vi "Handle Camera Configuration.vi"(9 "CameraNameRef":refnum<vi>, 10 "Display Name":string="Camera", 11 "ClusterRef":refnum<vi>) -> ()   [LabVIEW 2017]
uses:
  <vilib>/Rock Robotics/Network Tables/Make Table Operation.ctl
  <vilib>/Utility/config.llb/Read Key (String).vi
  <vilib>/Utility/config.llb/Read Key (I32).vi
  <vilib>/Utility/config.llb/Write Key (String).vi
  <vilib>/Utility/config.llb/Write Key (I32).vi
  <vilib>/Utility/config.llb/NI_LVConfig.lvlib
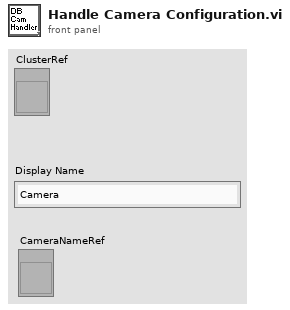
[diagram p1: front panel]
types:
  T1 = typedef "NI_LVConfig.lvlib/Config Data RefNum.ctl" = refnum<k1>
  T2 = cluster{"value":i32, "value":i32, "index":i32, bool}
  T3 = typedef "Make Table Operation.ctl" = enum16{"Get or Add Field", "Get Field or Add Temp", "Replace Temp ID", "Get Field ID - No Add", "Get Table Field IDs", "Get Field ID Info", "Move Field to Temp", "Validate", "Remove Field", "Remove All"}
  T4 = cluster{"Frame Rate":i32, "Compression":i32, "Size":u16, "DB Camera Config":bool}
  T5 = typedef "Field ID.ctl" = i32
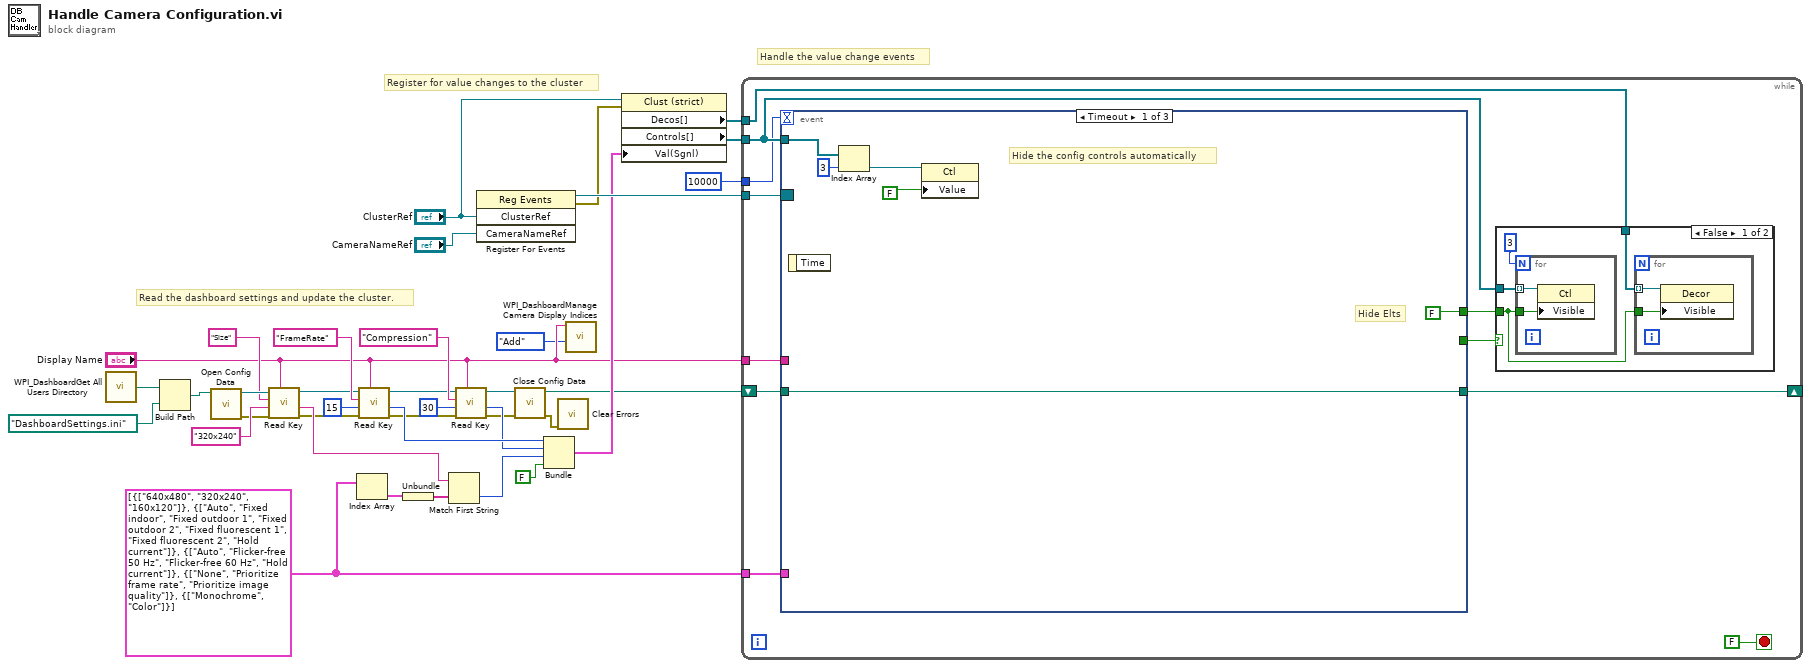
[diagram p0: block diagram]
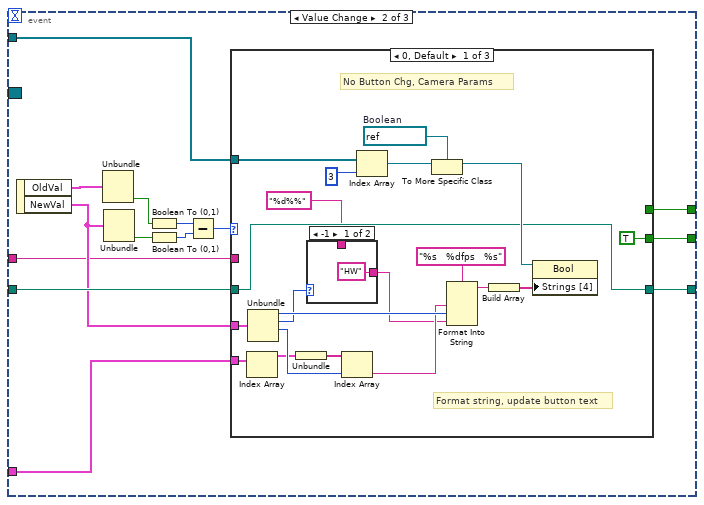
[diagram p3: hidden frame]
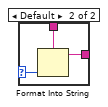
[diagram p4: hidden frame]
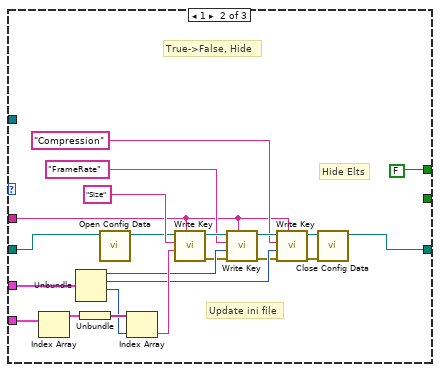
[diagram p5: hidden frame]
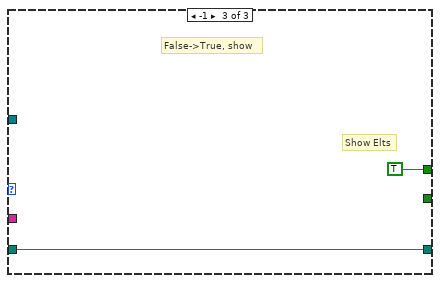
[diagram p6: hidden frame]
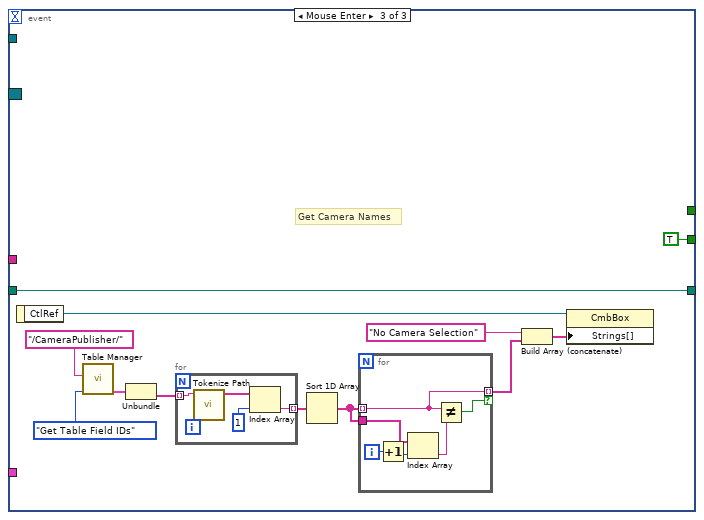
[diagram p7: hidden frame]
diagram:
  w16 = cluster{string[]}[] [{["640x480", "320x240", "160x120"]}, {["Auto", "Fixed indoor", "Fixed outdoor 1", "Fixed outdoor 2", "Fixed fluorescent 1", "Fixed fluorescent 2", "Hold current"]}, {["Auto", "Flicker-free 50 Hz", "Flicker-free 60 Hz", "Hold current"]}, {["None", "Prioritize frame rate", "Prioritize image quality"]}, {["Monochrome", "Color"]}]
  # "Handle the value change events"
  # "Register for value changes to the cluster"
  # "Read the dashboard settings and update the cluster."
  n1 = call <vilib>:"WPI_DashboardGet All Users Directory.vi"() -> ("All User Path"=w34:path)
  n2 = Build Path(base path=w34, name or relative path=path "DashboardSettings.ini") -> (appended path=w33:path)
  n3 = call <vilib>:"Open Config Data.vi"("configuration file path"=w33) -> ("error out"=w10:errorcluster, "refnum"=w32:T1)  [unwired: 8 in, 1 out]
  n4 = call-poly <vilib>:"Read Key.vi"("section"="Display Name", "error in (no error)"=w10, "default value"="320x240", "key"="Size", "refnum"=w32) -> ("error out"=w9:errorcluster, "value"=w20:string, "refnum out"=w24:T1)  [unwired: 1 in, 3 out]
  n5 = Index Array(array=w16) -> (element=w22:cluster{string[]})  [unwired: 1 in]
  n6 = call-poly <vilib>:"Read Key.vi"("section"="Display Name", "error in (no error)"=w9, "default value"=15, "key"="FrameRate", "refnum"=w24) -> ("error out"=w8:errorcluster, "value"=w18:i32, "refnum out"=w23:T1)  [unwired: 4 out]
  n7 = Unbundle(w22) -> (w21:string[])
  n8 = Match First String(2:w21, 3:w20) -> (0:w19:i32)  [unwired: 1 out]
  n9 = call-poly <vilib>:"Read Key.vi"("section"="Display Name", "error in (no error)"=w8, "default value"=30, "key"="Compression", "refnum"=w23) -> ("error out"=w5:errorcluster, "value"=w17:i32, "refnum out"=w7:T1)  [unwired: 4 out]
  n10 = register-events("ClusterRef", "CameraNameRef") -> (reference out=w37:refnum<event-registration>, error out=w14:errorcluster)  [unwired: 2 in]
  n11 = call <vilib>:"Close Config Data.vi"("error in (no error)"=w5, "refnum"=w7) -> ("error out"=w4:errorcluster, "file path"=w6:path)  [unwired: 1 in, 7 out]
  n12 = Bundle("value"=w18, "value"=w17, "index"=w19, FALSE) -> (w13:T2)  [unwired: 1 out]
  n13 = call <vilib>:"Clear Errors.vi"("error in (no error)"=w4) -> ()  [unwired: 5 in, 2 out]
  n14 = call <vilib>:"WPI_DashboardManage Camera Display Indices.vi"("Operation"=enum16{"Add", "Retrieve"}."Add", "Display Name"="Display Name") -> ()  [unwired: 9 in, 1 out]
  n15 = property class="Clust (strict)"(reference="ClusterRef", error in=w14, "Val(Sgnl)"=w13) -> ("Decos[]"=w12:refnum<vi>[], "Controls[]"=w35:refnum<vi>[])  [unwired: 2 out]
  n16 = while {
    tunnel: w37 -> [w48]
    tunnel: w35 -> [w40]
    shift-right: [w46] -> _
    shift-left: w6 -> [w47]
    tunnel: w16 -> [w45]
    tunnel: "Display Name" -> [w43]
    tunnel: w12 -> [w39]
    tunnel: 10000 -> [w38]
    stop <- FALSE stop-if-true
    n17 = event shown="[0] Timeout" {
      selector: w48 -> [_ _ _]
      dyn-events: _ -> [_ _ _]
      timeout: w38 -> [_ _ _]
      tunnel: w47 -> [w61 w70 w134]
      tunnel: [w61 w66 w134] -> w46
      tunnel: w45 -> [_ w68 _]
      tunnel: w40 -> [w60 w67 _]
      tunnel: w43 -> [_ w65 _]
      tunnel: [FALSE w64 _] -> w41
      tunnel: [_ w63 TRUE] -> w42
      event Timeout {
        # "Hide Elts"
        # "Hide the config controls automatically"
        n18 = event-data() -> ()  [unwired: 1 in, 1 out]
        n19 = Index Array(array=w60, index=3) -> (element=w58:refnum<vi>)
        n20 = property class="Ctl"(reference=w58, "Value"=FALSE) -> ()  [unwired: 1 in, 2 out]
      }
      event Value Change {
        n21 = event-data() -> ("OldVal"=w72:T4, "NewVal"=w69:T4)  [unwired: 1 in]
        n22 = Unbundle(w72) -> ("DB Camera Config"=w76:bool)  [unwired: 3 out]
        n23 = Unbundle(w69) -> ("DB Camera Config"=w75:bool)  [unwired: 3 out]
        n24 = Boolean To (0,1)(Boolean=w76) -> (0, 1=w73:i16)
        n25 = Boolean To (0,1)(Boolean=w75) -> (0, 1=w74:i16)
        n26 = Subtract(x=w73, y=w74) -> (x-y=w71:i16)
        n27 = case shown="0, Default" w71 {
          tunnel: [_ FALSE TRUE] -> w64
          tunnel: [TRUE _ _] -> w63
          tunnel: w70 -> [w80 w103 w123]
          tunnel: w69 -> [w88 w112 _]
          tunnel: w68 -> [w87 w108 _]
          tunnel: w67 -> [w86 _ _]
          tunnel: [w80 w101 w123] -> w66
          tunnel: w65 -> [_ w107 _]
          frame 0, Default {
            w83 = refnum<vi> refnum  # Boolean
            # "Format string, update button text"
            # "No Button Chg, Camera Params"
            n28 = Index Array(array=w87) -> (element=w91:cluster{string[]})  [unwired: 1 in]
            n29 = Unbundle(w88) -> ("Frame Rate"=w95:i32, "Compression"=w77:i32, "Size"=w93:u16)  [unwired: 1 out]
            n30 = Unbundle(w91) -> (w92:string[])
            n31 = case shown="-1" w77 {
              selector: w77 -> [_ w98]
              tunnel: "%d%%" ("format string") -> [_ w100]
              tunnel: ["HW" ("format string") w99] -> w78
              frame -1 {
              }
              frame Default {
                n32 = Format Into String(format string=w100, w98) -> (resulting string=w99:string)  [unwired: 2 in, 1 out]
              }
            }
            n33 = Index Array(array=w92, index=w93) -> (element=w94:string)
            n34 = Index Array(array=w86, index=3) -> (element=w84:refnum<vi>)
            n35 = To More Specific Class(target class=w83, reference=w84) -> (specific class reference=w82:refnum<vi>)  [unwired: 1 in, 1 out]
            n36 = Format Into String(format string="%s   %dfps   %s", w94, w95, w78) -> (resulting string=w90:string)  [unwired: 2 in, 1 out]
            n37 = Build Array(w90) -> (w81:string[])
            n38 = property class="Bool"(reference=w82, "Strings [4]"=w81) -> ()  [unwired: 1 in, 2 out]
          }
          frame 1 {
            # "Update ini file"
            # "Hide Elts"
            # "True->False, Hide"
            n39 = Index Array(array=w108) -> (element=w116:cluster{string[]})  [unwired: 1 in]
            n40 = Unbundle(w112) -> ("Frame Rate"=w111:i32, "Compression"=w110:i32, "Size"=w109:u16)  [unwired: 1 out]
            n41 = Unbundle(w116) -> (w115:string[])
            n42 = call <vilib>:"Open Config Data.vi"("configuration file path"=w103) -> ("refnum"=w102:T1)  [unwired: 8 in, 2 out]
            n43 = Index Array(array=w115, index=w109) -> (element=w114:string)
            n44 = call-poly <vilib>:"Write Key.vi"("section"=w107, "value"=w114, "key"="Size", "refnum"=w102) -> ("error out"=w106:errorcluster, "refnum out"=w121:T1)  [unwired: 2 in, 4 out]
            n45 = call-poly <vilib>:"Write Key.vi"("section"=w107, "error in (no error)"=w106, "value"=w111, "key"="FrameRate", "refnum"=w121) -> ("error out"=w105:errorcluster, "refnum out"=w120:T1)  [unwired: 5 out]
            n46 = call-poly <vilib>:"Write Key.vi"("section"=w107, "error in (no error)"=w105, "value"=w110, "key"="Compression", "refnum"=w120) -> ("error out"=w104:errorcluster, "refnum out"=w113:T1)  [unwired: 5 out]
            n47 = call <vilib>:"Close Config Data.vi"("error in (no error)"=w104, "refnum"=w113) -> ("file path"=w101:path)  [unwired: 1 in, 8 out]
          }
          frame -1 {
            # "Show Elts"
            # "False->True, show"
          }
        }
      }
      event Mouse Enter {
        # "Get Camera Names"
        n48 = event-data() -> ("CtlRef"=w136:refnum<vi>)  [unwired: 1 in]
        n49 = call <vilib>:"Table Manager.vi"("Operation"=Make_Table_Operation."Get Table Field IDs", "Entry Name"="/CameraPublisher/") -> ("Entries"=w131:cluster{"Entry IDs":T5[], "Names":string[]})  [unwired: 6 in, 3 out]
        n50 = Unbundle(w131) -> ("Names"=w128:string[])  [unwired: 1 out]
        n51 = for {
          tunnel: w128 -> [w146] mode=indexing
          tunnel: [w143] -> w127 mode=indexing
          n52 = call <vilib>:"Tokenize Path.vi"("Name"=w146) -> ("Array"=w145:string[])  [unwired: 10 in]
          n53 = Index Array(array=w145, index=1) -> (element=w143:string)
        }
        n54 = Sort 1D Array(array=w127) -> (sorted array=w126:string[])
        n55 = for {
          tunnel: w126 -> [w138] mode=indexing
          tunnel: w126 -> [w140]
          tunnel: [w138] -> w125 mode=indexing if=w137
          i -> [w142]
          n56 = Increment(x=w142) -> (x+1=w141:i32)
          n57 = Index Array(array=w140, index=w141) -> (element=w139:string)
          n58 = Not Equal?(x=w138, y=w139) -> (x != y?=w137:bool)
        }
        n59 = Build Array (concatenate)("No Camera Selection", w125) -> (w129:string[])
        n60 = property class="CmbBox"(reference=w136, "Strings[]"=w129) -> ()  [unwired: 1 in, 2 out]
      }
    }
    n61 = case shown="False" w42 {
      tunnel: w40 -> [w52 _]
      tunnel: w41 -> [w49 _]
      tunnel: w39 -> [w50 _]
      frame False {
        n62 = for {
          N: 3 -> [_]
          tunnel: w52 -> [w56] mode=indexing
          tunnel: w49 -> [w55]
          n63 = property class="Ctl"(reference=w56, "Visible"=w55) -> ()  [unwired: 1 in, 2 out]
        }
        n64 = for {
          tunnel: w50 -> [w54] mode=indexing
          tunnel: w49 -> [w53]
          n65 = property class="Decor"(reference=w54, "Visible"=w53) -> ()  [unwired: 1 in, 2 out]
        }
      }
      frame True {
      }
    }
  }
